vi "DisplayLogic_DrawBlockMask.vi"(2 "ActivePixel":cluster{"h_pixel":i16, "v_pixel":i16}) -> (16 "PixelData":bool[](array[boolean]))   [LabVIEW 2018]
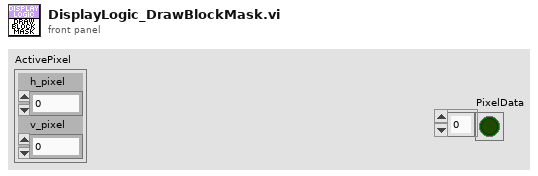
[diagram p1: front panel]
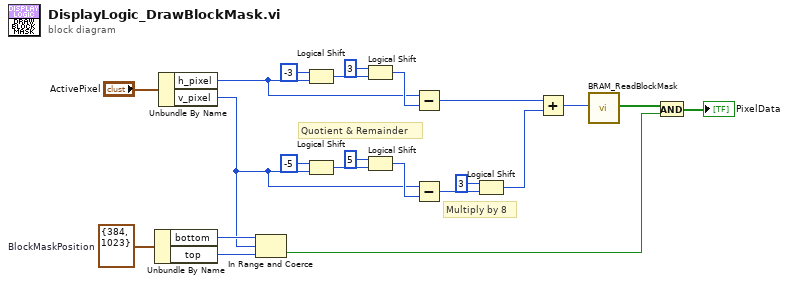
[diagram p0: block diagram]
diagram:
  w1 = cluster{"top":i16, "bottom":i16} {"top"=384, "bottom"=1023}  # BlockMaskPosition
  # "Quotient & Remainder"
  # "Multiply by 8"
  n1 = Unbundle By Name(w1) -> ("bottom"=w7:i16, "top"=w6:i16)
  n2 = Unbundle By Name("ActivePixel") -> ("h_pixel"=w3:i16, "v_pixel"=w2:i16)
  n3 = In Range and Coerce(upper limit=w7, x=w2, lower limit=w6) -> (In Range?=w5:bool)  [unwired: 1 out]
  n4 = Logical Shift(y=i16 -3, x=w3) -> (x << y=w10:i16)
  n5 = Logical Shift(y=i16 -5, x=w2) -> (x << y=w17:i16)
  n6 = Logical Shift(y=i16 3, x=w10) -> (x << y=w11:i16)
  n7 = Logical Shift(y=i16 5, x=w17) -> (x << y=w16:i16)
  n8 = Subtract(x=w3, y=w11) -> (x-y=w4:i16)
  n9 = Subtract(x=w2, y=w16) -> (x-y=w14:i16)
  n10 = Logical Shift(y=i16 3, x=w14) -> (x << y=w13:i16)
  n11 = Add(x=w4, y=w13) -> (x+y=w12:i16)
  n12 = call "BRAM_ReadBlockMask.vi"("Address"=w12) -> ("PixelData"=w21:bool[])  [unwired: 18 in]
  n13 = And(x=w21, y=w5) -> (x .and. y?=→"PixelData":bool[])
